vi "Shared Variables CD 2.0 Main Page.vi"(8 "error in (no error)":errorcluster, 11 "Node Ptr":T1 format="%.0x") -> (0 "error out":errorcluster)   [LabVIEW 2017, in "Shared Variables CD 2.0 Configuration.lvlib"]
uses:
  Shared Variables CD 2.0 Configuration.lvlib
  <vilib>/NI Veristand/Custom Device API/Custom Device Item Ref.ctl
  Shared/SV Global.vi
  <vilib>/NI VeriStand/Custom Device API/Custom Device API.lvlib
panel:
  out "Version":string
  in  "Update rate (ms)":dbl=10.0 min=0.001 step=0.001
  in  "Info":refnum<k7>(container)
  in  "Header":cluster{"Section Name":string}={"Section Name"="Custom Device Item Settings"}
  in  "Description":string
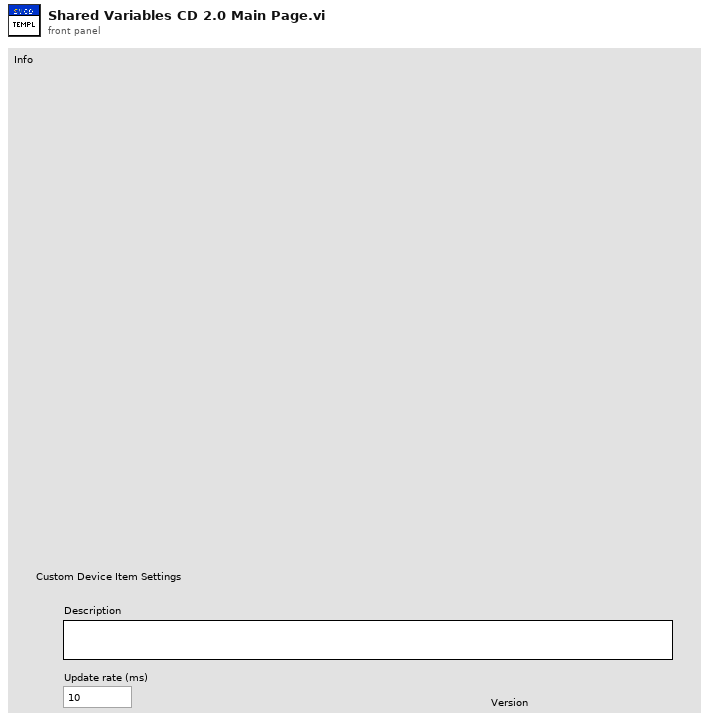
[diagram p1: front panel]
types:
  T1 = typedef "Custom Device API.lvlib/Custom Device Item Ref.ctl" = u64
  T2 = typedef "Custom Device API.lvlib/Custom Device Commands.ctl" = enum16{"Default", "Item renamed", "Shutdown", "Dynamic button pressed"}
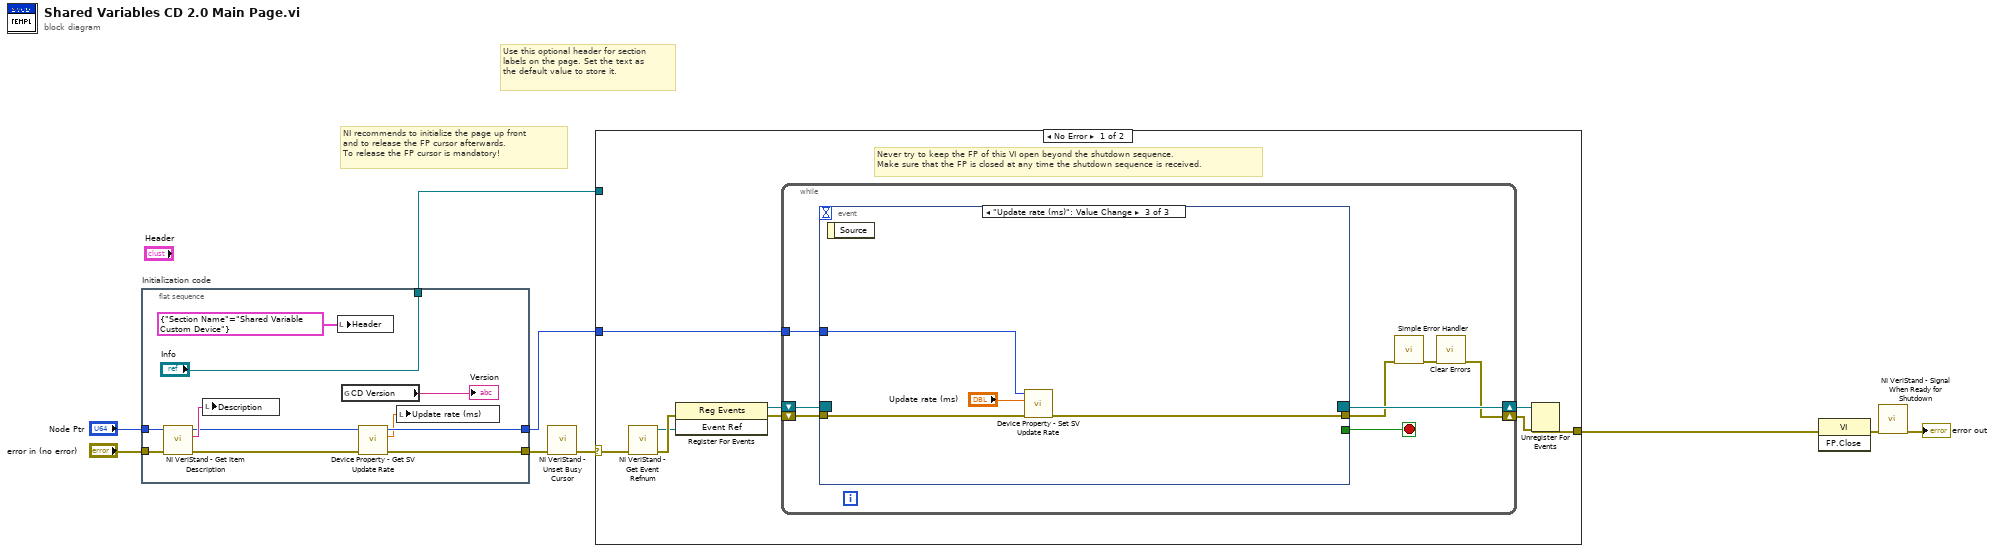
[diagram p0: block diagram]
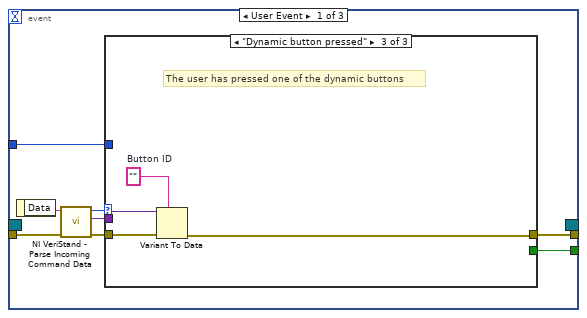
[diagram p2: hidden frame]
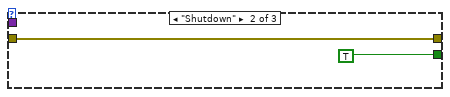
[diagram p4: hidden frame]
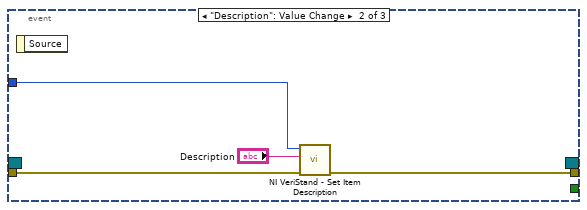
[diagram p5: hidden frame]
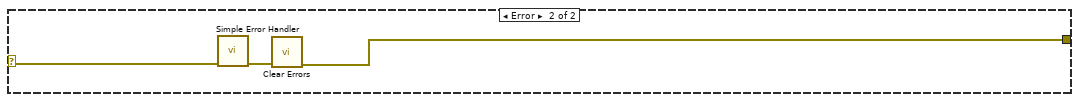
[diagram p6: hidden frame]
diagram:
  # "Use this optional header for section labels on the page. Set the text as the default value to store it."
  # "NI recommends to initialize the page up front\nand to release the FP cursor afterwards.\nTo release the FP cursor is mandatory!"
  n1 = flat-sequence "Initialization code" {
    tunnel: "error in (no error)" -> [w20]
    tunnel: "Node Ptr" -> [w19]
    tunnel: [w12] -> w3
    tunnel: ["Info"] -> w2
    tunnel: [w13] -> w1
    frame #0 {
      n2 = call <vilib>:"NI VeriStand - Get Item Description.vi"("error in (no error)"=w20, "Item Ref in"=w19) -> ("error out"=w14:errorcluster, "Description"=w18:string, "Item Ref out"=w15:T1)  [unwired: 7 out]
      n3 = local write "Description"(w18) -> ()
      n4 = local write "Header"(cluster{"Section Name":string} {"Section Name"="Shared Variable Custom Device"} ("Header")) -> ()
      n5 = global read "SV Global.vi" "CD Version"() -> (→"Version":string)
      n6 = call "Device Property - Get SV Update Rate.vi"("error in (no error)"=w14, "Device Ref in"=w15) -> ("error out"=w13:errorcluster, "Update Rate (ms)"=w11:dbl, "Device Ref out"=w12:T1)  [unwired: 7 in]
      n7 = local write "Update rate (ms)"(w11) -> ()
    }
  }
  n8 = call <vilib>:"NI VeriStand - Unset Busy Cursor.vi"("error in (no error)"=w1) -> ("error out"=w5:errorcluster)  [unwired: 10 out]
  n9 = case shown="No Error" w5 {
    selector: w5 -> [w21 w63]
    tunnel: [w26 w61] -> w9
    tunnel: w3 -> [w22 _]
    tunnel: w2 -> [_ _]
    frame No Error {
      # "Never try to keep the FP of this VI open beyond the shutdown sequence.\nMake sure that the FP is closed at any time the shutdown sequence is received."
      n10 = call <vilib>:"NI VeriStand - Get Event Refnum.vi"("error in (no error)"=w21) -> ("error out"=w29:errorcluster, "Event Ref"=w25:refnum<user-event>)  [unwired: 9 out]
      n11 = register-events(error in=w29, w25) -> (reference out=w23:refnum<event-registration>, error out=w24:errorcluster)  [unwired: 1 in]
      n12 = while {
        tunnel: w22 -> [w33]
        shift-right: [w30] -> w27
        shift-left: w24 -> [w36]
        shift-right: [w37] -> w28
        shift-left: w23 -> [w35]
        stop <- w34 stop-if-true
        n13 = event shown="[2] \"Update rate (ms)\": Value Change" {
          selector: w35 -> [_ _ _]
          dyn-events: [_ _ _] -> w37
          timeout: _ -> [_ _ _]
          tunnel: w36 -> [w45 w55 w58]
          tunnel: [w41 _ _] -> w34
          tunnel: [w40 w54 w57] -> w32
          tunnel: w33 -> [w39 w56 w60]
          event User Event {
            n14 = event-data() -> ("Data"=w44:string)  [unwired: 1 out]
            n15 = call <vilib>:"NI VeriStand - Parse Incoming Command Data.vi"("error in (no error)"=w45, "Incoming data"=w44) -> ("error out"=w43:errorcluster, "Outgoing data"=w38:variant, "Action"=w42:T2)  [unwired: 7 out]
            n16 = case shown="\"Dynamic button pressed\"" w42 {
              tunnel: w43 -> [w46 w47 w52]
              tunnel: [_ TRUE _] -> w41
              tunnel: [w46 w47 w49] -> w40
              tunnel: w39 -> [_ _ _]
              tunnel: w38 -> [_ _ w51]
              frame "Default", Default {
              }
              frame "Shutdown" {
              }
              frame "Dynamic button pressed" {
                w50 = ""  # Button ID
                # "The user has pressed one of the dynamic buttons"
                n17 = Variant To Data(error in=w52, type=w50, Variant=w51) -> (error out=w49:errorcluster)  [unwired: 1 out]
              }
            }
          }
          event "Description": Value Change {
            n18 = event-data() -> ()  [unwired: 2 out]
            n19 = call <vilib>:"NI VeriStand - Set Item Description.vi"("error in (no error)"=w55, "Description"="Description", "Item Ref in"=w56) -> ("error out"=w54:errorcluster)  [unwired: 8 out]
          }
          event "Update rate (ms)": Value Change {
            n20 = event-data() -> ()  [unwired: 2 out]
            n21 = call "Device Property - Set SV Update Rate.vi"("error in (no error)"=w58, "Update Rate (ms)"="Update rate (ms)", "Device Ref in"=w60) -> ("error out"=w57:errorcluster)  [unwired: 7 in, 1 out]
          }
        }
        n22 = call <vilib>:"Simple Error Handler.vi"("error in (no error)"=w32) -> ("error out"=w31:errorcluster)  [unwired: 1 in, 7 out]
        n23 = call <vilib>:"Clear Errors.vi"("error in (no error)"=w31) -> ("error out"=w30:errorcluster)  [unwired: 1 in, 5 out]
      }
      n24 = Unregister For Events(event registration refnum=w28, error in=w27) -> (error out=w26:errorcluster)
    }
    frame Error {
      n25 = call <vilib>:"Simple Error Handler.vi"("error in (no error)"=w63) -> ("error out"=w62:errorcluster)  [unwired: 1 in, 7 out]
      n26 = call <vilib>:"Clear Errors.vi"("error in (no error)"=w62) -> ("error out"=w61:errorcluster)  [unwired: 1 in, 5 out]
    }
  }
  n27 = invoke class="VI" method="FP.Close"(error in=w9) -> (error out=w8:errorcluster)  [unwired: 2 in, 2 out]
  n28 = call <vilib>:"NI VeriStand - Signal When Ready for Shutdown.vi"("error in (no error)"=w8) -> ("error out"=→"error out":errorcluster)  [unwired: 10 out]
